vi "Write Bus Access.vi"(8 "error in (no error)":errorcluster, 10 "Var Access":refnum<class "Bus_Access.lvclass">[](array[class]), 11 "Var Bus in":refnum<class "Omni_Bus.lvclass">) -> (0 "error out":errorcluster, 3 "Var Bus out":refnum<class "Omni_Bus.lvclass">)   [LabVIEW 2021, in "Omni_Bus.lvclass"]
uses:
  Omni_Bus.lvclass
  Bus Access/Bus_Access.lvclass
  Omni_Bus.lvclass/Omni_Bus.ctl
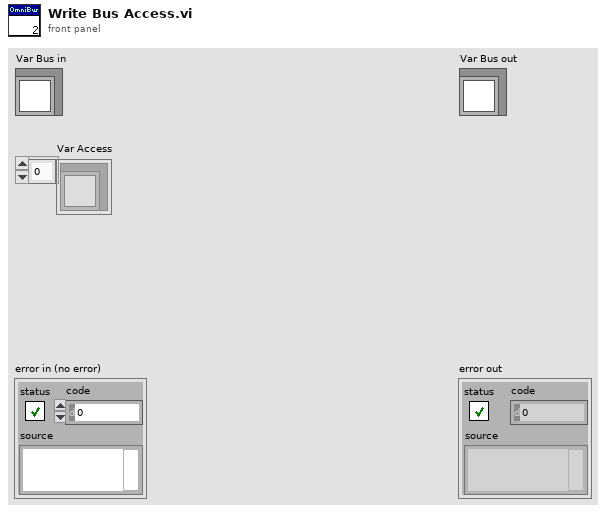
[diagram p1: front panel]
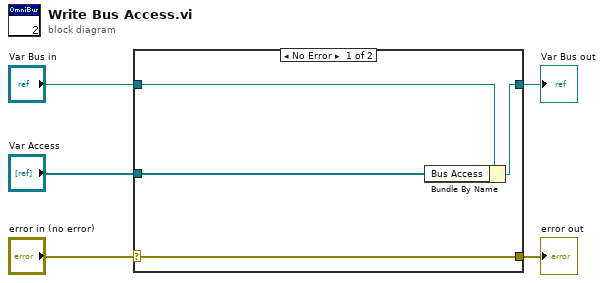
[diagram p0: block diagram]
diagram:
  n1 = case shown="No Error" "error in (no error)" {
    selector: "error in (no error)" -> [w9 w10]
    tunnel: [w9 w10] -> w4
    tunnel: [w7 w11] -> w2
    tunnel: "Var Bus in" -> [w8 w11]
    tunnel: "Var Access" -> [w6 _]
    frame No Error {
      n2 = Bundle By Name(cluster=w8, "Bus Access"=w6) -> (w7:refnum<class "Omni_Bus.lvclass">)
    }
    frame Error {
    }
  }
  "error out" <- w4
  "Var Bus out" <- w2
